vi "Close.vi"() -> ()   [LabVIEW 2017, in "SVPWMInterface.lvlib"]
uses:
  SVPWMInterface.lvlib
  SVPWMInterface.ctl
  <instrlib>/_niInstr/Instruction Framework/v1/Host/Instruction Target/niInstr Instruction Target v1 Host.lvclass
  <instrlib>/_niInstr/Instruction Framework/v1/Host/Instruction Framework Context/niInstr Instruction Framework Context v1 Host.lvclass
panel:
  out "error out":errorcluster
  in  "error in":errorcluster
  in  "Interface":T1
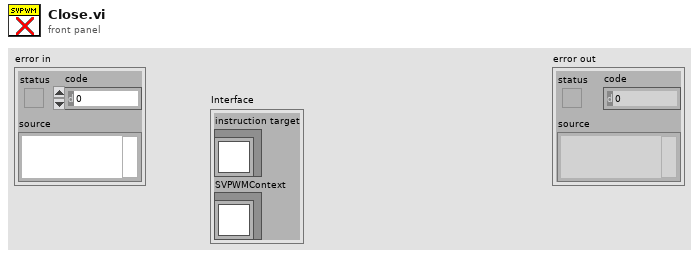
[diagram p1: front panel]
types:
  T1 = typedef "SVPWMInterface.lvlib/SVPWMInterface.ctl" = cluster{"instruction target":refnum<class "niInstr Instruction Target v1 Host.lvclass">, "SVPWMContext":refnum<class "niInstr Instruction Framework Context v1 Host.lvclass">}
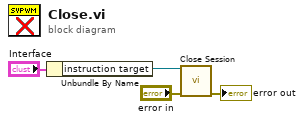
[diagram p0: block diagram]
diagram:
  n1 = Unbundle By Name("Interface") -> ("instruction target"=w3:refnum<class "niInstr Instruction Target v1 Host.lvclass">)
  n2 = call-dynamic "Close Session.vi"("instruction target"=w3, "error in"="error in") -> ("error out"=→"error out":errorcluster)  [unwired: 13 in]
